vi "APU and ECU Control.vi"(8 "error in (no error)":errorcluster, 11 "APU & ECU Control":T1) -> (0 "error out":errorcluster)   [LabVIEW 2018, in "PC UDP Writer.lvlib"]
doc: "This subVI enqueues the named action in to the communications queue along with the input data."
uses:
  PC UDP Writer.lvlib
  Testing UI 1/Private Controls/APU & ECU Controls.ctl
  Private Controls/Module Data.ctl
  Private Controls/Module Action.ctl
  Testing UI 1/Testing UI 1.lvlib
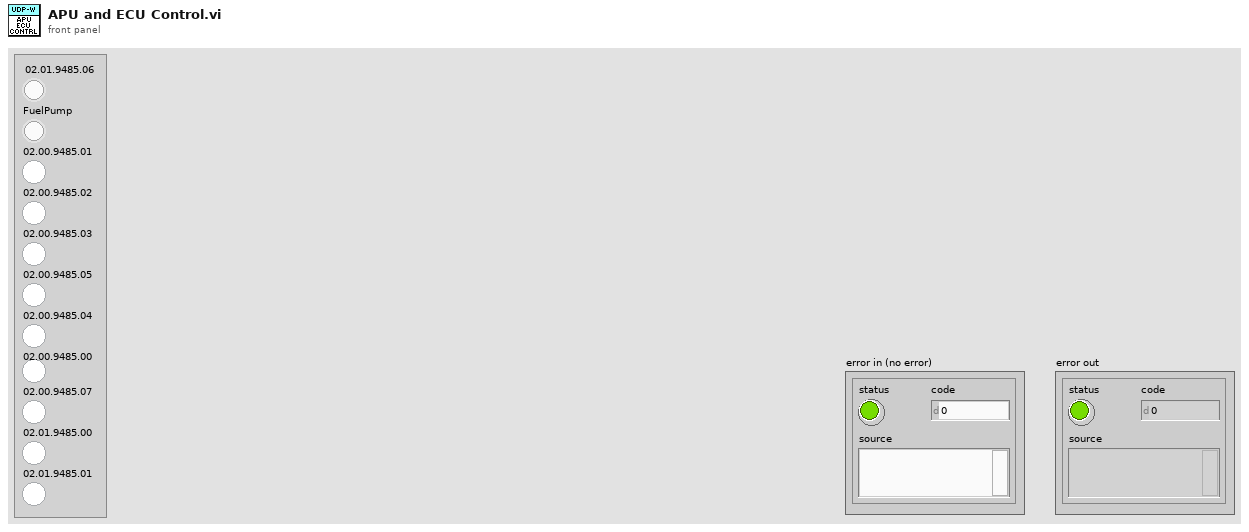
[diagram p1: front panel]
types:
  T1 = typedef "Testing UI 1.lvlib/APU & ECU Controls.ctl" = cluster{"02.01.9485.06":bool, "FuelPump":bool, "02.00.9485.01":bool, "02.00.9485.02":bool, "02.00.9485.03":bool, "02.00.9485.05":bool, "02.00.9485.04":bool, "02.00.9485.00":bool, "02.00.9485.07":bool, "02.01.9485.00":bool, "02.01.9485.01":bool}
  T2 = typedef "PC UDP Writer.lvlib/Module Data.ctl" = cluster{"Data":variant, "Action":T3}
  T3 = typedef "PC UDP Writer.lvlib/Module Action.ctl" = enum8{"Init", "Waterfall Select", "Bleed Fuel", "Fuel Pressure Reg", "ECS Demand", "Accel Sensitivities", "Accel Filters", "Shunt Relay", "APU Setup", "APU and ECU Control", "APU Start", "Write", "Error", "Exit"}
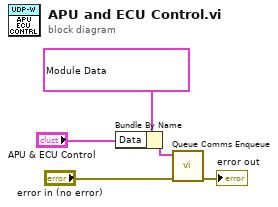
[diagram p0: block diagram]
diagram:
  n1 = Bundle By Name(cluster=T2 {"Data"=variant, "Action"=enum."APU and ECU Control"} ("element"), "Data"="APU & ECU Control") -> (w2:T2)
  n2 = call "Queue Comms Enqueue.vi"("error in (no error)"="error in (no error)", "element"=w2) -> ("error out"=→"error out":errorcluster)  [unwired: 9 in]
